vi "Open Turret Subsystem.vi"() -> (14 "CAN Talon SRX Ref":T3={"DeviceStatus"={"status"=FALSE, "code"=0, "source"=""}, "Type"=enum."PWM", "PWM"={"PWM Channel"=enum."Invalid", "DeadBand"={"Name"="", "maxPositivePwm"=0, "minPositivePwm"=0, "centerPwm"=0, "maxNegativePwm"=0, "minNegativePwm"=0, "angularRange"=0}}, "CAN"={"Device Number"=0, "Control Mode"=enum."Percent VBus", "Semaphore"=refnum, "Max Vout"=12.0, "TalonSRX Control Mode"=enum."Percent VBus"}, "Invert"=FALSE}, 15 "navX Device":T1={"Interface"={"Protocol"=enum."SERIAL", "Update Rate (4Hz-60Hz)"=4, "navX Open TypeDef"=variant}, "Notify Packet"=refnum, "Loop VI Refnum"=refnum, "Ready to Close Occurrence Refnum"=refnum} {"Interface"."Update Rate (4Hz-60Hz)" min=4 max=60 step=1}, 16 "dead zone":dbl, 17 "motor error out":errorcluster, 19 "navX error out":errorcluster)   [LabVIEW 2015]
uses:
  <vilib>/Rock Robotics/WPI/MotorControl/WPI_MotorControlDeviceRef.ctl
  <vilib>/Rock Robotics/WPI/MotorControl/WPI_MotorControlType.ctl
  <vilib>/Rock Robotics/SystemInterfaces/DIO/FPGA_DIOPWMChannel.ctl
  <vilib>/Rock Robotics/WPI/PWM/WPI_PWMDeadband.ctl
  <vilib>/Rock Robotics/WPI/CAN/Jaguar/SubVIs/WPI_CANJaguar_ControlMode.ctl
  <vilib>/Rock Robotics/WPI/CAN/TalonSRX/WPI_CANTalonSRX_APIControlMode.ctl
  Support Code/navX Library v2/Z900_navX_DeviceTypeDef.ctl
  Support Code/navX Library v2/Z900_navX_ProtocolTypeDef.ctl
  Support Code/navX Library v2/Z900_navX_NotifyPacketTypeDef.ctl
  Support Code/navX Library v2/Z900_navX_ActionTypeDef.ctl
  <vilib>/Rock Robotics/WPI/CAN/TalonSRX/WPI_CANTalonSRX_APIFeedbackSelect.ctl
  <vilib>/Rock Robotics/WPI/MotorControl/WPI_MotorControlOpenCANTalonSRX.vi
  Support Code/navX Library v2/navX Library v2.lvlib
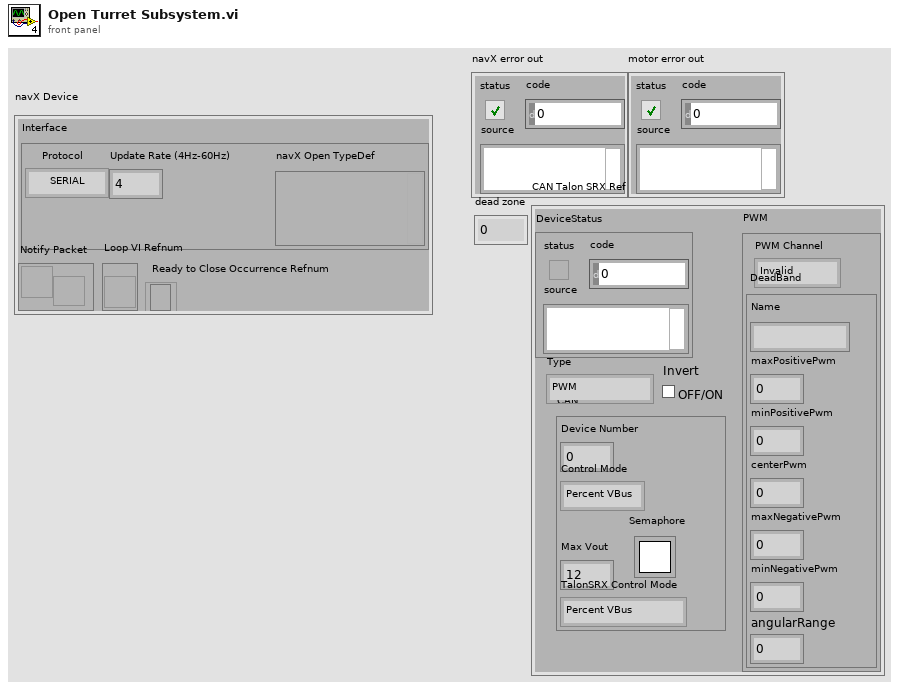
[diagram p1: front panel]
types:
  T1 = typedef "navX Library v2.lvlib/Z900_navX_DeviceTypeDef.ctl" = cluster{"Interface":cluster{"Protocol":T2, "Update Rate (4Hz-60Hz)":u8, "navX Open TypeDef":variant}, "Notify Packet":refnum<notifier>, "Loop VI Refnum":refnum<vi>, "Ready to Close Occurrence Refnum":refnum<k4>}
  T2 = typedef "navX Library v2.lvlib/Z900_navX_ProtocolTypeDef.ctl" = enum16{"SERIAL", "I2C", "SPI"}
  T3 = typedef "WPI_MotorControlDeviceRef.ctl" = cluster{"DeviceStatus":errorcluster, "Type":T4, "PWM":cluster{"PWM Channel":T5, "DeadBand":T6}, "CAN":cluster{"Device Number":u8, "Control Mode":T7, "Semaphore":T8, "Max Vout":dbl, "TalonSRX Control Mode":T9}, "Invert":bool}
  T4 = typedef "WPI_MotorControlType.ctl" = enum16{"PWM", "CAN", "CANTalonSRX"}
  T5 = typedef "FPGA_DIOPWMChannel.ctl" = enum8{"PWM 0", "PWM 1", "PWM 2", "PWM 3", "PWM 4", "PWM 5", "PWM 6", "PWM 7", "PWM 8", "PWM 9", "PWM MXP 0", "PWM MXP 1", "PWM MXP 2", "PWM MXP 3", "PWM MXP 4", "PWM MXP 5", "PWM MXP 6", "PWM MXP 7", "PWM MXP 8", "PWM MXP 9", "Invalid"}
  T6 = typedef "WPI_PWMDeadband.ctl" = cluster{"Name":string, "maxPositivePwm":i32, "minPositivePwm":i32, "centerPwm":i32, "maxNegativePwm":i32, "minNegativePwm":i32, "angularRange":u16}
  T7 = typedef "WPI_CANJaguar_ControlMode.ctl" = enum8{"Percent VBus", "Current", "Speed", "Position", "Voltage"}
  T8 = typedef "Semaphore RefNum" = refnum<k1>
  T9 = typedef "WPI_CANTalonSRX_APIControlMode.ctl" = enum8{"Percent VBus", "Speed", "Position", "Slave", "Unchanged / Invalid", "Voltage Compensation", "Current", "Motion Profile"}
  T10 = typedef "WPI_CANTalonSRX_APIFeedbackSelect.ctl" = enum16{"Digital Quadrature Encoder", "Analog Potentiometer", "Analog Encoder", "Count on Quad-A (Rising-Edge)", "Count on Quad-A (Falling-Edge)", "CTR Magnetic Enc (Absolute)", "CTR Magnetic Enc (Relative)", "Pulse Width"}
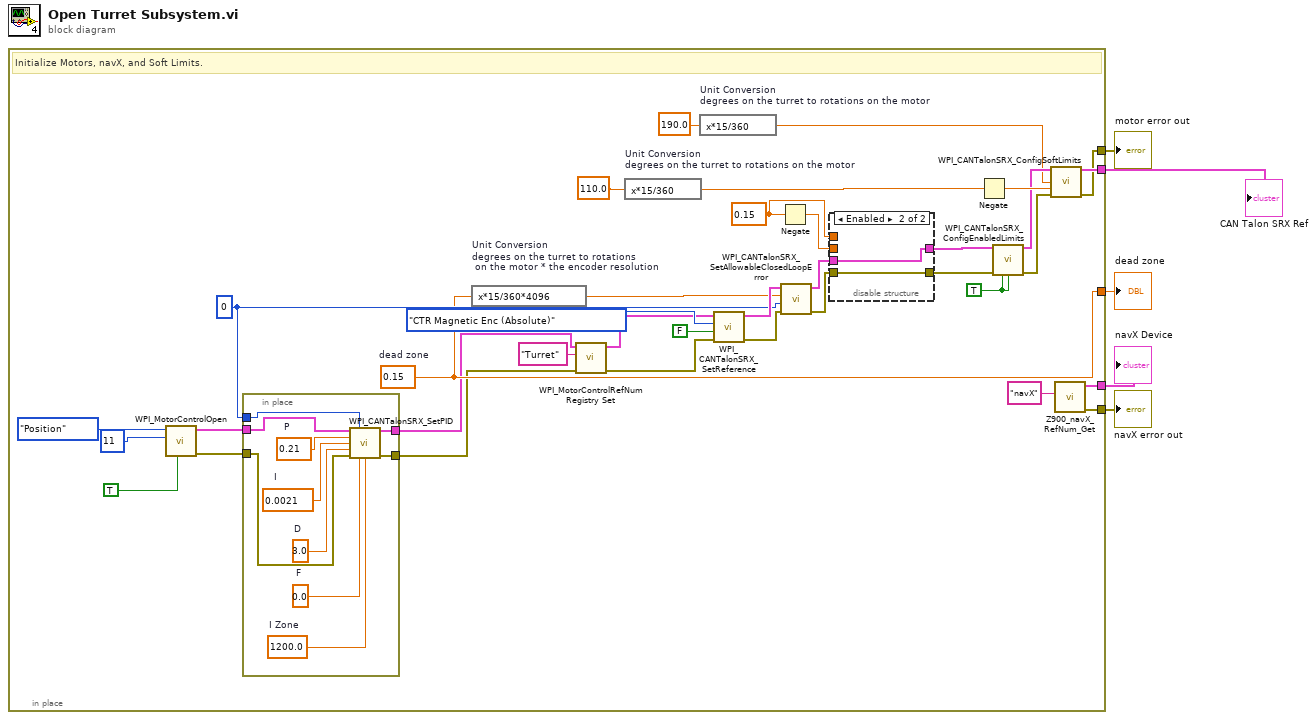
[diagram p0: block diagram]
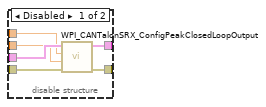
[diagram p2: hidden frame]
diagram:
  n1 = in-place {
    in-place-border: [w35] -> w2
    in-place-border: [w34] -> w4
    in-place-border: [w32] -> w5
    in-place-border: [w31] -> w1
    in-place-border: [w14] -> w3
    w17 = 0.15
    w14 = 0.15  # dead zone
    w18 = u8 0 ("Parameter Slot")
    w21 = TRUE ("Forward Soft Limit Enable")
    # "Initialize Motors, navX, and Soft Limits."
    n2 = call-poly <vilib>:"WPI_MotorControlOpen.vi"("Invert"=TRUE, "Device Number"=11, "Control Mode"=WPI_CANTalonSRX_APIControlMode."Position") -> ("error out"=w38:errorcluster, "MotorControlDeviceRef"=w39:T3)  [unwired: 7 in]
    n3 = in-place {
      in-place-border: w39 -> [w59]
      in-place-border: w38 -> [w58]
      in-place-border: [w50] -> w8
      in-place-border: [w51] -> w10
      in-place-border: w18 -> [w52]
      w53 = 1200.0  # I Zone
      w54 = 0.0  # F
      w55 = 3.0  # D
      w56 = 0.0021  # I
      w57 = 0.21  # P
      n4 = call <vilib>:"WPI_CANTalonSRX_SetPID.vi"("CAN Talon SRX Ref"=w59, "Parameter Slot"=w52, "P"=w57, "I"=w56, "D"=w55, "error in (no error)"=w58, "F"=w54, "I Zone"=w53) -> ("CAN Talon SRX Ref"=w51:T3, "error out"=w50:errorcluster)  [unwired: 6 in]
    }
    n5 = expression code="x*15/360*4096" "Unit Conversion\ndegrees on the turret to rotations\n on the motor * the encoder resolution"(w14) -> (w13:dbl)
    n6 = call <vilib>:"WPI_MotorControlRefNum Registry Set.vi"("error in (no error)"=w8, "refnum name"="Turret", "MotorControlDevRef"=w10) -> ("error out"=w7:errorcluster, "MotorControlDevRef"=w9:T3)  [unwired: 7 in]
    n7 = expression code="x*15/360" "Unit Conversion\ndegrees on the turret to rotations on the motor"(110.0 ("Forward Limit Position")) -> (w29:dbl)
    n8 = expression code="x*15/360" "Unit Conversion\ndegrees on the turret to rotations on the motor"(190.0 ("Forward Limit Position")) -> (w11:dbl)
    n9 = call <vilib>:"WPI_CANTalonSRX_SetReference.vi"("error in (no error)"=w7, "Reverse Feedback Sensor"=FALSE, "Feedback Reference"=WPI_CANTalonSRX_APIFeedbackSelect."CTR Magnetic Enc (Absolute)", "CAN Talon SRX Ref"=w9) -> ("error out"=w27:errorcluster, "CAN Talon SRX Ref"=w26:T3)  [unwired: 6 in]
    n10 = Negate(x=w17) -> (-x=w16:dbl)
    n11 = call <vilib>:"WPI_CANTalonSRX_SetAllowableClosedLoopError.vi"("error in (no error)"=w27, "Parameter Slot"=w18, "Allowable Closed-Loop Error"=w13, "CAN Talon SRX Ref"=w26) -> ("error out"=w25:errorcluster, "CAN Talon SRX Ref"=w24:T3)  [unwired: 6 in]
    n12 = disable-structure shown="Enabled" {
      disable-tunnel: w25 -> [w47 w48]
      disable-tunnel: w24 -> [w46 w49]
      disable-tunnel: [w45 w49] -> w23
      disable-tunnel: [w44 w48] -> w22
      disable-tunnel: w17 -> [w43 _]
      disable-tunnel: w16 -> [w42 _]
      frame Disabled {
        n13 = call <vilib>:"WPI_CANTalonSRX_ConfigPeakClosedLoopOutput.vi"("error in (no error)"=w47, "Reverse Peak Output"=w42, "Forward Peak Output"=w43, "CAN Talon SRX Ref"=w46) -> ("error out"=w44:errorcluster, "CAN Talon SRX Ref"=w45:T3)  [unwired: 6 in]
      }
      frame Enabled {
      }
    }
    n14 = Negate(x=w29) -> (-x=w28:dbl)
    n15 = call <vilib>:"WPI_CANTalonSRX_ConfigEnabledLimits.vi"("CAN Talon SRX Ref"=w23, "error in (no error)"=w22, "Forward Soft Limit Enable"=w21, "Reverse Soft Limit Enable"=w21) -> ("CAN Talon SRX Ref"=w19:T3, "error out"=w20:errorcluster)  [unwired: 10 in]
    n16 = call <vilib>:"WPI_CANTalonSRX_ConfigSoftLimits.vi"("CAN Talon SRX Ref"=w19, "Forward Limit Position"=w11, "Reverse Limit Position"=w28, "error in (no error)"=w20) -> ("CAN Talon SRX Ref"=w35:T3, "error out"=w34:errorcluster)  [unwired: 10 in]
    n17 = call "Z900_navX_RefNum_Get.vi"("refnum name"="navX") -> ("error out"=w32:errorcluster, "navX Device"=w31:T1)  [unwired: 9 in]
  }
  "navX error out" <- w5
  "motor error out" <- w4
  "dead zone" <- w3
  "CAN Talon SRX Ref" <- w2
  "navX Device" <- w1
